vi "Add Ports and Sections.vi"(8 "error in":errorcluster, 10 "board configuration in":T1 {"portConfiguration"."Rx_UDP"."Tx_UDP"."FilterMode" items=["FDX_RX_VL_FLT_DIS", "FDX_RX_VL_FLT_ENA ", "FDX_RX_VL_FLT_ENA_INV"]; "portConfiguration"."Rx_UDP"."Tx_UDP"."VLBufSize" format="%.0x"; "portConfiguration"."Rx_UDP"."Tx_UDP"."VerificationMode" items=["FDX_RX_VL_CHECK_ENA_DEFAULT"=65535, "FDX_RX_VL_CHECK_REDMAM"=16, "DX_RX_VL_CHECK_TRAFIC"=8, "FDX_RX_VL_CHECK_FRAMESIZE"=4, "FDX_RX_VL_CHECK_SNINTEG"=2, "FDX_RX_VL_CHECK_INVPAC"=1, "FDX_RX_VL_CHECK_DISA"=0]; "portConfiguration"."Tx_UDP"."tx_udp_setup"."interfaceID" format="%.0b"; "portConfiguration"."Tx_UDP"."tx_udp_setup"."NetSelect" items=["FDX_TX_FRAME_DLY_A"=0, "FDX_TX_FRAME_DLY_B"=1, "FDX_TX_FRAME_BOTH "=3, "FDX_TX_FRAME_ONLY_A"=4, "FDX_TX_FRAME_ONLY_B "=5]; "portConfiguration"."Rx_Monitor"."Strobe" items=["FDX_MON_STROBE_DIS", "FDX_MON_STROBE_STOP", "FDX_MON_STROBE_START"]; "portConfiguration"."Rx_Monitor"."CaptureMode" items=["FDX_MON_SINGLE ", "FDX_MON_CONTINUOUS", "FDX_MON_SELECTIVE", "FDX_MON_RECORDING", "FDX_MON_REROS", "FDX_MON_HMU"]; "portConfiguration"."Rx_Monitor"."DefaultCronoMode" items=["FDX_RX_DEFAULT_ENA_CNT", "FDX_RX_DEFAULT_MON_ENA_ALL", "FDX_RX_DEFAULT_MON_ENA_GOOD"]; "portConfiguration"."Tx_Generic"."Frame Headers"."Frame header"."PhysErrorInjection" items=["FDX_TX_FRAME_ERR_OFF", "FDX_TX_FRAME_ERR_CRC", "FDX_TX_FRAME_ERR_ALI", "FDX_TX_FRAME_ERR_PRE", "FDX_TX_FRAME_ERR_PHY"]; "portConfiguration"."Tx_Generic"."Frame Headers"."Frame header"."PayloadGenerationMode" items=["FDX_TX_FRAME_PGM_USER", "FDX_TX_FRAME_PGM_IP_PART", "FDX_TX_FRAME_PGM_IP_PART_TT", "FDX_TX_FRAME_PGM_IP_FULL", "FDX_TX_FRAME_PGM_IP_FULL_TT"]; "portConfiguration"."Tx_Generic"."Frame Headers"."Frame header"."PayloadBufferMode" items=["FDX_TX_FRAME_PBM_STD", "FDX_TX_FRAME_PBM_MAC", "FDX_TX_FRAME_PBM_UDP", "FDX_TX_FRAME_PBM_FULL"]; "portConfiguration"."Tx_Generic"."Frame Headers"."Frame header"."NetSelect" items=["FDX_TX_FRAME_DLY_A"=0, "FDX_TX_FRAME_DLY_B"=1, "FDX_TX_FRAME_BOTH "=3, "FDX_TX_FRAME_ONLY_A"=4, "FDX_TX_FRAME_ONLY_B "=5]; "portConfiguration"."Tx_Generic"."Frame Headers"."Frame header"."FrameStartMode" items=["FDX_TX_FRAME_START_IFG", "FDX_TX_FRAME_START_PGWT", "FDX_TX_FRAME_START_TRG", "FDX_TX_FRAME_START_TRG_D"]; "portConfiguration"."Tx_Generic"."tx_generic_setup"."StartMode" items=["FDX_STOP", "FDX_START", "FDX_START_TRG", "FDX_START_TIME"]; "boardSetup"."portConfig" items=["FDX_SINGLE", "FDX_REDUNDANT"]; "boardSetup"."portSpeed" items=["FDX_100MBIT", "FDX_10MBIT", "FDX_AUTO_100MBIT", "FDX_AUTO_10MBIT", "FDX_AUTO_ERROR", "FDX_1000MBIT"]}, 11 "custom device ref":T18=18446744073709551615 format="%.0x") -> (0 "error out":errorcluster, 3 "custom device ref out":T18=18446744073709551615 format="%.0x")   [LabVIEW 2020, in "AIM ARINC 664 Scripting.lvlib"]
uses:
  AIM ARINC 664 Scripting.lvlib
  <vilib>/NI VeriStand/Custom Device API/Custom Device Item Ref.ctl
  Import/_typedefs/Board Top Level Configuration.ctl
  Import/_typedefs/board_setup.ctl
  Import/_typedefs/port_configuration.ctl
  Import/_typedefs/port_setup.ctl
  Import/_typedefs/session_tx_generic.ctl
  Import/_typedefs/tx_generic_setup.ctl
  Import/_typedefs/frame_tx_generic.ctl
  Import/_typedefs/frame_tx_generic_seqNumberInit.ctl
  Import/_typedefs/frame_tx_generic_seqNumberOffset.ctl
  Import/_typedefs/frame_parameter.ctl
  Import/_typedefs/frame_parameter_definition.ctl
  Shared/Encoding (Arinc664).ctl
  Import/_typedefs/port_tx_udp_comm.ctl
  Import/_typedefs/port_tx_udp_sap.ctl
  Import/_typedefs/rx_udp_setup.ctl
  Import/_typedefs/port_rx_udp_comm.ctl
  Import/_typedefs/port_rx_udp_sap.ctl
  <vilib>/NI/VeriStand Custom Device Serialization/System Explorer Action.ctl
  <vilib>/NI VeriStand/Custom Device API/Custom Device API.lvlib
  <vilib>/NI/VeriStand Custom Device Serialization/Custom Device Serialization.lvlib
  Import/AIM ARINC 664 Import.lvlib
panel:
  # "This Control below has Typedefs removed because it was creating a crash in LV 2020 SP1. If we do not support his version, we should try to use the cluster with Typedefs."
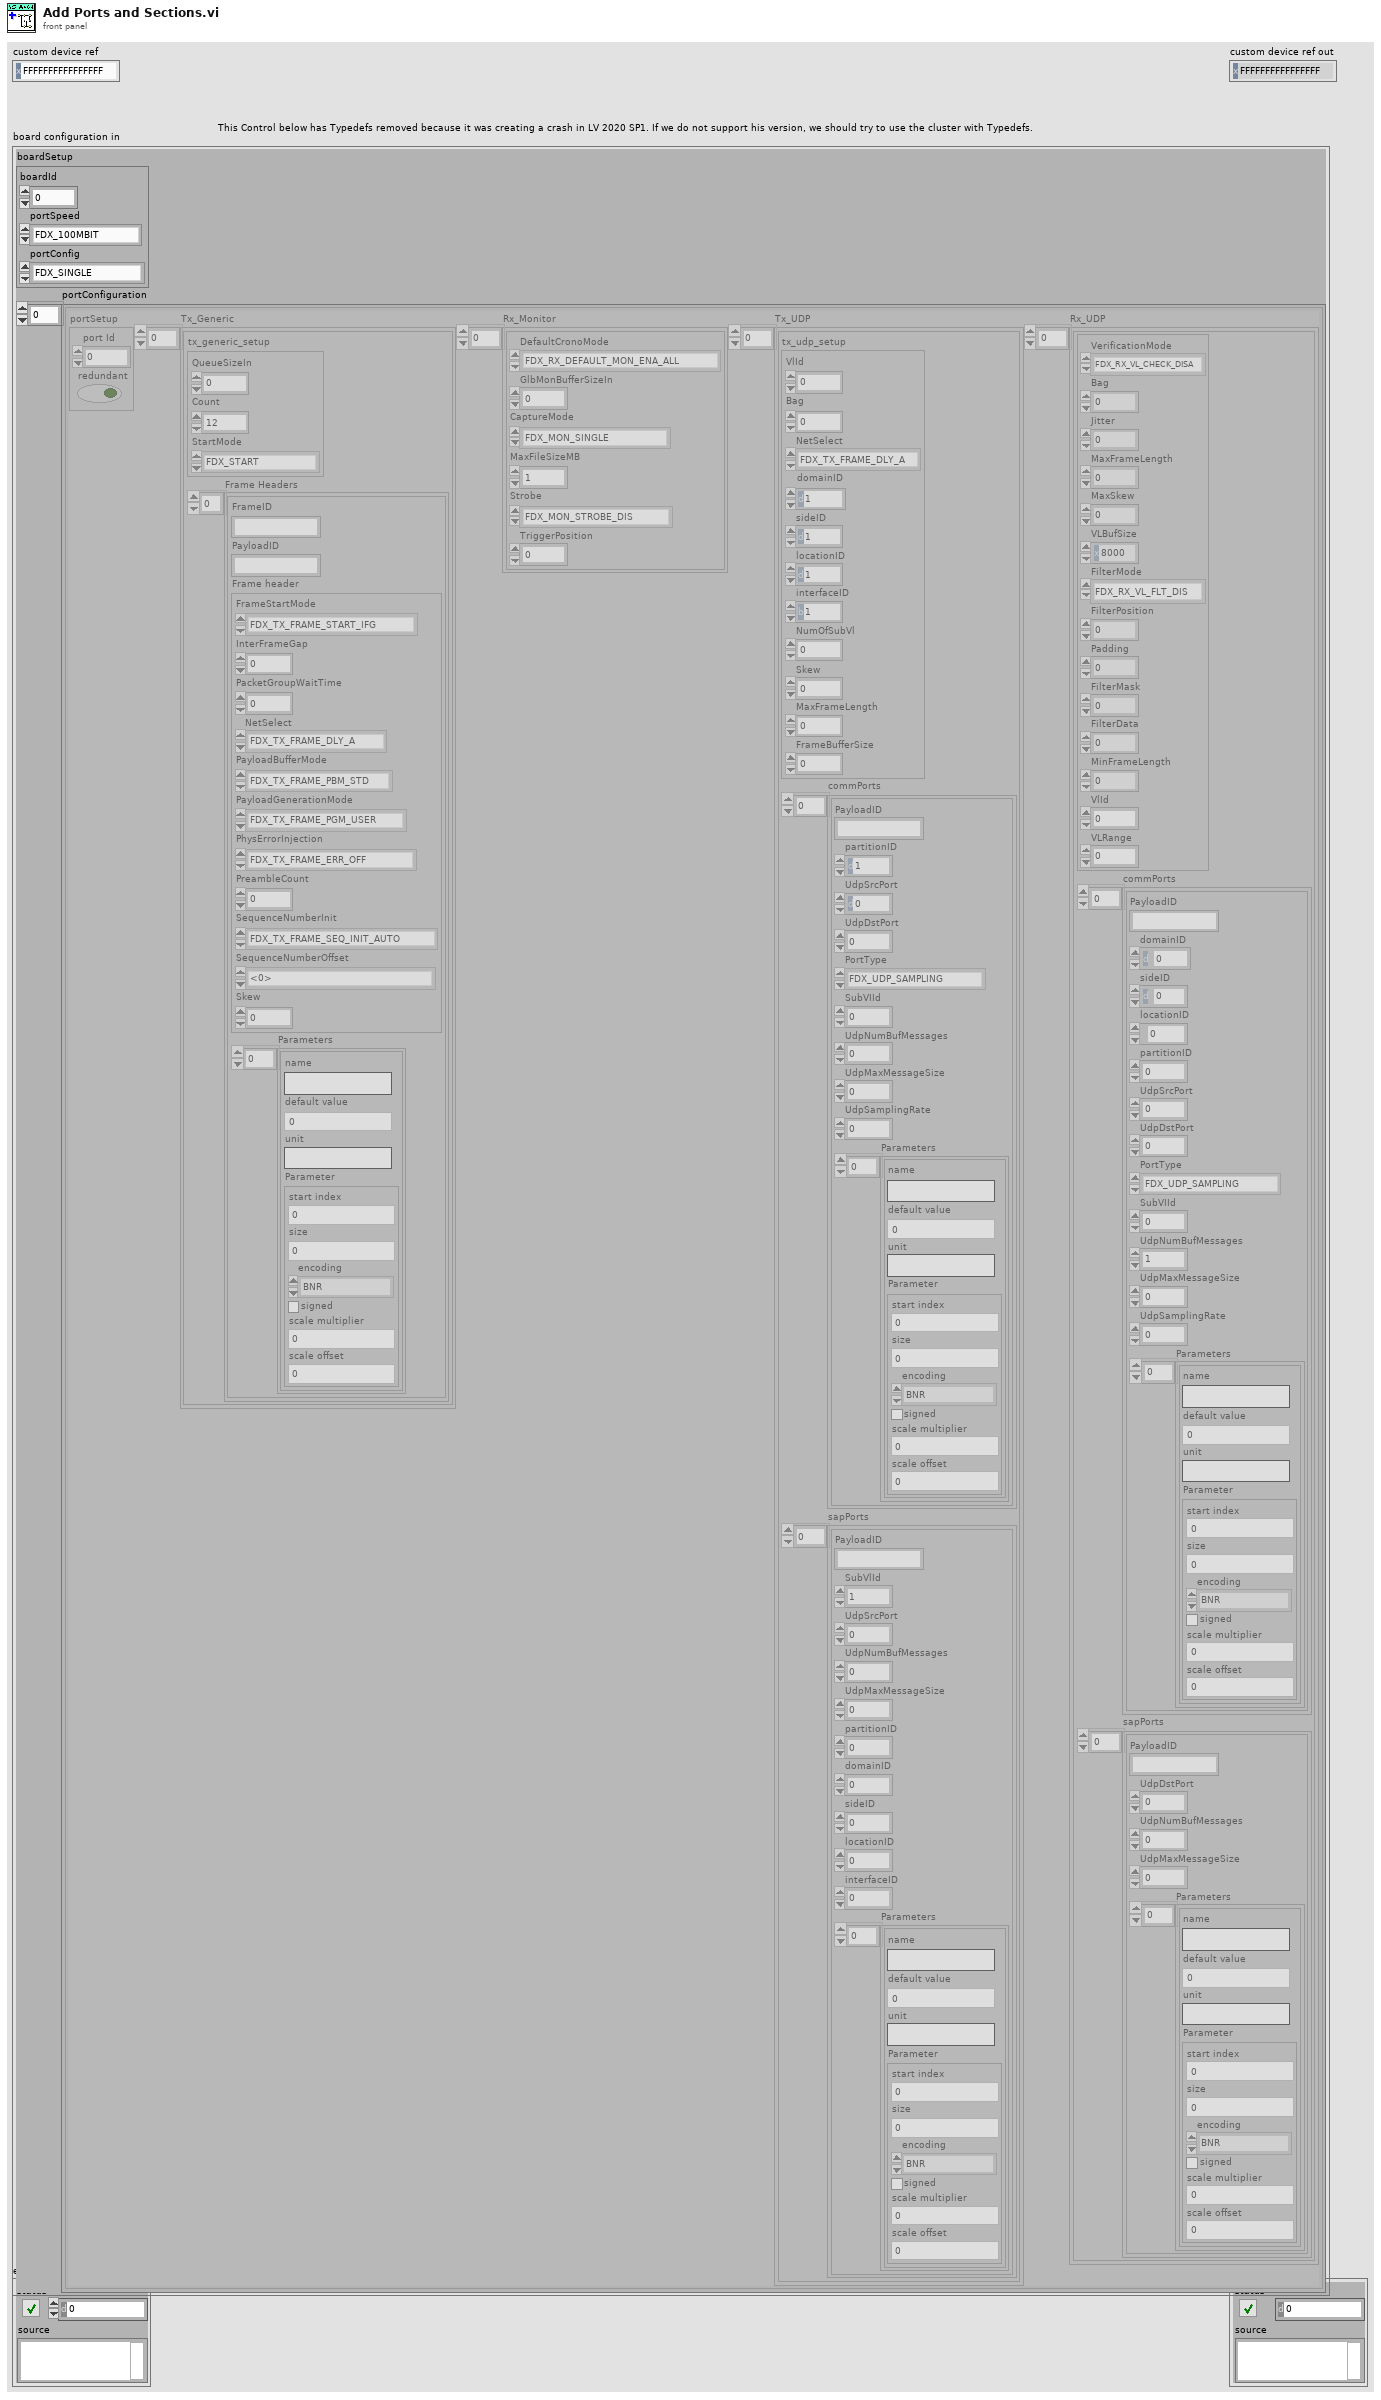
[diagram p1: front panel]
types:
  T1 = typedef "AIM ARINC 664 Import.lvlib/Board Top Level Configuration.ctl" = cluster{"boardSetup":T2, "portConfiguration":T3[]}
  T2 = typedef "AIM ARINC 664 Import.lvlib/board_setup.ctl" = cluster{"boardId":u32, "portSpeed":u32, "portConfig":u32}
  T3 = typedef "AIM ARINC 664 Import.lvlib/port_configuration.ctl" = cluster{"portSetup":T4, "Tx_Generic":T5[], "Rx_Monitor":cluster{"DefaultCronoMode":u32, "GlbMonBufferSizeIn":u32, "CaptureMode":u32, "MaxFileSizeMB":u32, "Strobe":u32, "TriggerPosition":u32}[], "Tx_UDP":cluster{"tx_udp_setup":cluster{"VlId":i32, "Bag":i32, "NetSelect":u32, "domainID":u8, "sideID":u8, "locationID":u8, "interfaceID":u8, "NumOfSubVl":u16, "Skew":u32, "MaxFrameLength":u32, "FrameBufferSize":u32}, "commPorts":T13[], "sapPorts":T14[]}[], "Rx_UDP":cluster{"Tx_UDP":T15, "commPorts":T16[], "sapPorts":T17[]}[]}
  T4 = typedef "AIM ARINC 664 Import.lvlib/port_setup.ctl" = cluster{"port Id":u32, "redundant":bool}
  T5 = typedef "AIM ARINC 664 Import.lvlib/session_tx_generic.ctl" = cluster{"tx_generic_setup":T6, "Frame Headers":T7[]}
  T6 = typedef "AIM ARINC 664 Import.lvlib/tx_generic_setup.ctl" = cluster{"QueueSizeIn":u32, "Count":i32, "StartMode":i32}
  T7 = typedef "AIM ARINC 664 Import.lvlib/frame_tx_generic.ctl" = cluster{"FrameID":string, "PayloadID":string, "Frame header":cluster{"FrameStartMode":i32, "InterFrameGap":i32, "PacketGroupWaitTime":i32, "NetSelect":u32, "PayloadBufferMode":i32, "PayloadGenerationMode":i32, "PhysErrorInjection":i32, "PreambleCount":i32, "SequenceNumberInit":T8, "SequenceNumberOffset":T9, "Skew":i32}, "Parameters":T10[]}
  T8 = typedef "AIM ARINC 664 Import.lvlib/frame_tx_generic_seqNumberInit.ctl" = i32
  T9 = typedef "AIM ARINC 664 Import.lvlib/frame_tx_generic_seqNumberOffset.ctl" = i32
  T10 = typedef "AIM ARINC 664 Import.lvlib/frame_parameter.ctl" = cluster{"name":string, "default value":dbl, "unit":string, "Parameter":T11}
  T11 = typedef "AIM ARINC 664 Import.lvlib/frame_parameter_definition.ctl" = cluster{"start index":i32, "size":i32, "encoding":T12, "signed":bool, "scale multiplier":dbl, "scale offset":dbl}
  T12 = typedef "Encoding (Arinc664).ctl" = u16
  T13 = typedef "AIM ARINC 664 Import.lvlib/port_tx_udp_comm.ctl" = cluster{"PayloadID":string, "partitionID":u8, "UdpSrcPort":u16, "UdpDstPort":u16, "PortType":enum16{"FDX_UDP_SAMPLING", "FDX_UDP_QUEUING"}, "SubVIId":u32, "UdpNumBufMessages":u32, "UdpMaxMessageSize":u32, "UdpSamplingRate":u32, "Parameters":T10[]}
  T14 = typedef "AIM ARINC 664 Import.lvlib/port_tx_udp_sap.ctl" = cluster{"PayloadID":string, "SubVlId":u8, "UdpSrcPort":u16, "UdpNumBufMessages":u32, "UdpMaxMessageSize":u32, "partitionID":u8, "domainID":u8, "sideID":u8, "locationID":u8, "interfaceID":u8, "Parameters":T10[]}
  T15 = typedef "AIM ARINC 664 Import.lvlib/rx_udp_setup.ctl" = cluster{"VerificationMode":u32, "Bag":u32, "Jitter":u32, "MaxFrameLength":u32, "MaxSkew":u32, "VLBufSize":u32, "FilterMode":u32, "FilterPosition":u32, "Padding":u32, "FilterMask":u32, "FilterData":u32, "MinFrameLength":u32, "VlId":u16, "VLRange":u32}
  T16 = typedef "AIM ARINC 664 Import.lvlib/port_rx_udp_comm.ctl" = cluster{"PayloadID":string, "domainID":u8, "sideID":u8, "locationID":u8, "partitionID":u8, "UdpSrcPort":u16, "UdpDstPort":u16, "PortType":enum16{"FDX_UDP_SAMPLING", "FDX_UDP_QUEUING"}, "SubVIId":u32, "UdpNumBufMessages":u32, "UdpMaxMessageSize":u32, "UdpSamplingRate":u32, "Parameters":T10[]}
  T17 = typedef "AIM ARINC 664 Import.lvlib/port_rx_udp_sap.ctl" = cluster{"PayloadID":string, "UdpDstPort":u16, "UdpNumBufMessages":u32, "UdpMaxMessageSize":u32, "Parameters":T10[]}
  T18 = typedef "Custom Device API.lvlib/Custom Device Item Ref.ctl" = u64
  T19 = typedef "Custom Device Serialization.lvlib/System Explorer Action.ctl" = u16
  T20 = cluster{"DefaultCronoMode":u32, "GlbMonBufferSizeIn":u32, "CaptureMode":u32, "MaxFileSizeMB":u32, "Strobe":u32, "TriggerPosition":u32}[]
  T21 = cluster{"tx_udp_setup":cluster{"VlId":i32, "Bag":i32, "NetSelect":u32, "domainID":u8, "sideID":u8, "locationID":u8, "interfaceID":u8, "NumOfSubVl":u16, "Skew":u32, "MaxFrameLength":u32, "FrameBufferSize":u32}, "commPorts":T13[], "sapPorts":T14[]}[]
  T22 = cluster{"Tx_UDP":T15, "commPorts":T16[], "sapPorts":T17[]}[]
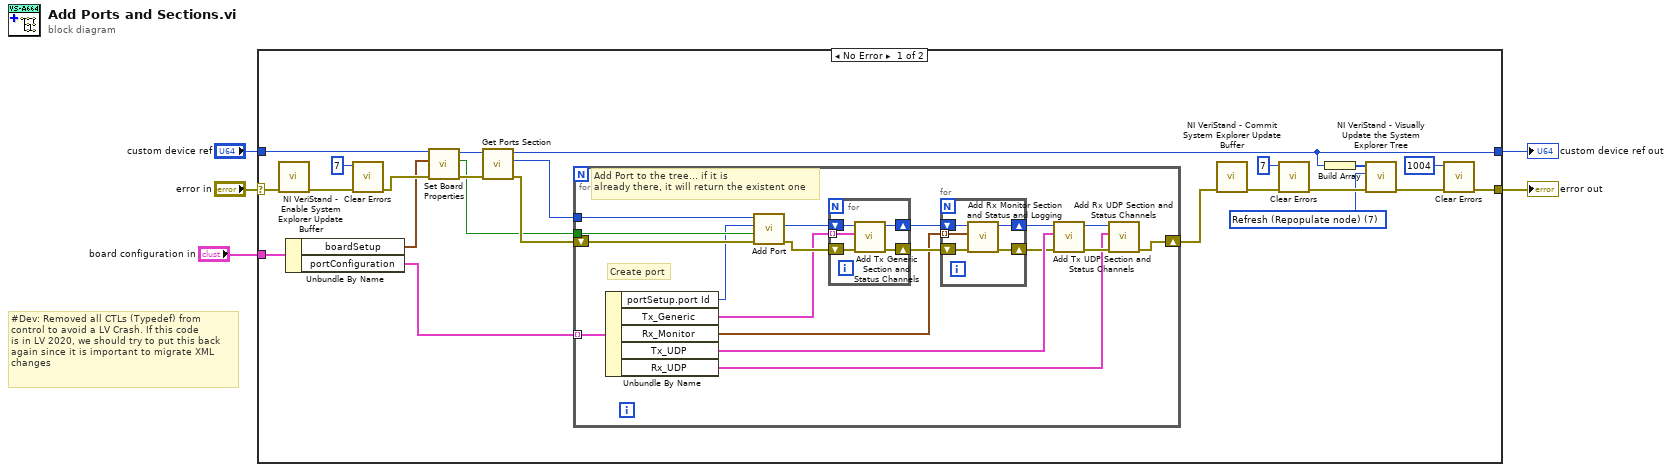
[diagram p0: block diagram]
diagram:
  # "#Dev: Removed all CTLs (Typedef) from\ncontrol to avoid a LV Crash. If this code\nis in LV 2020, we should try to put this back\nagain since it is important to migrate XML\nchanges"
  n1 = case shown="No Error" "error in" {
    selector: "error in" -> [w28 w58]
    tunnel: "custom device ref" -> [w14 w57]
    tunnel: [w18 w58] -> w3
    tunnel: [w11 w57] -> w2
    tunnel: "board configuration in" -> [w6 _]
    frame No Error {
      w20 = T19 7 items=["Refresh (Add)"=5, "Refresh (Repopulate node)"=7] ("Action")
      n2 = call <vilib>:"NI VeriStand - Enable System Explorer Update Buffer.vi"("error in (no error)"=w28) -> ("error out"=w26:errorcluster)  [unwired: 10 in]
      n3 = Unbundle By Name(w6) -> ("boardSetup"=w12:T2, "portConfiguration"=w7:T3[])
      n4 = call <vilib>:"Clear Errors.vi"("error in (no error)"=w26, "specific error code to clear (0: all)"=7) -> ("error out"=w13:errorcluster)  [unwired: 4 in, 1 out]
      n5 = call "Set Board Properties.vi"("error in"=w13, "board setup"=w12, "custom device ref in"=w14) -> ("error out"=w16:errorcluster, "redundant?"=w8:bool, "custom device ref out"=w15:T18)  [unwired: 6 in]
      n6 = call "Get Ports Section.vi"("error in"=w16, "custom device ref"=w15) -> ("error out"=w27:errorcluster, "ports ref out"=w10:T18, "custom device ref out"=w11:T18)  [unwired: 6 in, 1 out]
      n7 = for {
        tunnel: w10 -> [w45]
        tunnel: w8 -> [w42]
        shift-right: [w46] -> w9
        shift-left: w27 -> [w43]
        tunnel: w7 -> [w44] mode=indexing
        # "Add Port to the tree... if it is \nalready there, it will return the existent one"
        # "Create port"
        n8 = Unbundle By Name(w44) -> ("portSetup.port Id"=w29:u32, "Tx_Generic"=w31:T5[], "Rx_Monitor"=w30:T20, "Tx_UDP"=w41:T21, "Rx_UDP"=w38:T22)
        n9 = call "Add Port.vi"("error in"=w43, "redundant ?"=w42, "port Id"=w29, "ports ref"=w45) -> ("error out"=w34:errorcluster, "port ref out"=w37:T18)  [unwired: 5 in, 1 out]
        n10 = for {
          tunnel: w31 -> [w47] mode=indexing
          shift-right: [w49] -> w33
          shift-left: w34 -> [w51]
          shift-right: [w48] -> w36
          shift-left: w37 -> [w50]
          n11 = call "Add Tx Generic Section and Status Channels.vi"("error in"=w51, "Tx generic configuration"=w47, "port ref"=w50) -> ("error out"=w49:errorcluster, "port ref out"=w48:T18)  [unwired: 7 in]
        }
        n12 = for {
          tunnel: w30 -> [w52] mode=indexing
          shift-right: [w55] -> w35
          shift-left: w36 -> [w54]
          shift-right: [w56] -> w32
          shift-left: w33 -> [w53]
          n13 = call "Add Rx Monitor Section and Status and Logging.vi"("error in"=w53, "session_rx_monitor"=w52, "port ref"=w54) -> ("error out"=w56:errorcluster, "port ref out"=w55:T18)  [unwired: 7 in]
        }
        n14 = call "Add Tx UDP Section and Status Channels.vi"("error in"=w32, "Tx UDP configuration"=w41, "port ref"=w35) -> ("error out"=w40:errorcluster, "port ref out"=w39:T18)  [unwired: 7 in]
        n15 = call "Add Rx UDP Section and Status Channels.vi"("error in"=w40, "Rx UDP configuration"=w38, "port ref"=w39) -> ("error out"=w46:errorcluster)  [unwired: 7 in, 1 out]
      }
      n16 = call <vilib>:"NI VeriStand - Commit System Explorer Update Buffer.vi"("error in (no error)"=w9) -> ("error out"=w24:errorcluster)  [unwired: 10 in]
      n17 = call <vilib>:"Clear Errors.vi"("error in (no error)"=w24, "specific error code to clear (0: all)"=7) -> ("error out"=w23:errorcluster)  [unwired: 4 in, 1 out]
      n18 = Build Array(w11) -> (w19:T18[])
      n19 = call <vilib>:"NI VeriStand - Visually Update the System Explorer Tree.vi"("error in (no error)"=w23, "Action"=w20, "Node IDs"=w19) -> ("error out"=w21:errorcluster)  [unwired: 8 in]
      n20 = call <vilib>:"Clear Errors.vi"("error in (no error)"=w21, "specific error code to clear (0: all)"=1004) -> ("error out"=w18:errorcluster)  [unwired: 4 in, 1 out]
    }
    frame Error {
    }
  }
  "error out" <- w3
  "custom device ref out" <- w2
